vi "Add Multiple Entries.vi"(8 "error in (no error)":errorcluster, 9 "Values":variant[](array[variant]) caption="Data", 10 "Keys":string[](array[string]) caption="Names", 11 "Registry in":refnum<class "Registry.lvclass">) -> (0 "error out":errorcluster, 2 "Replaced?":bool[](array[boolean]), 3 "Registry out":refnum<class "Registry.lvclass">)   [LabVIEW 2020, in "BCI-1553 API.lvlib" / "Registry.lvlib" / "Registry.lvclass"]
doc: "Adds multiple Key/Value pairs to the Registry."
uses:
  Registry.lvclass
  Registry.lvclass/Registry.ctl
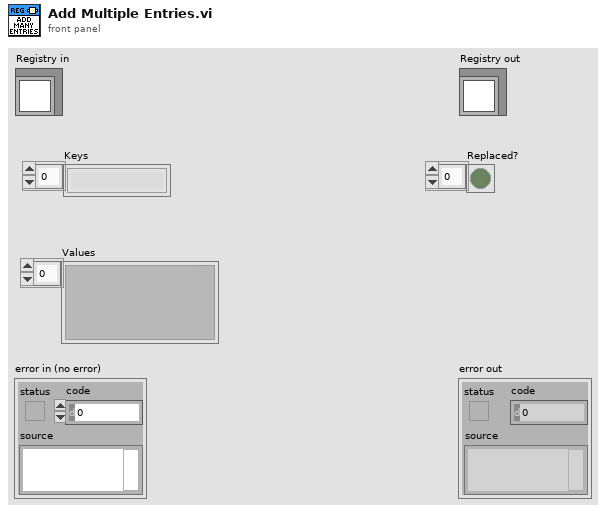
[diagram p1: front panel]
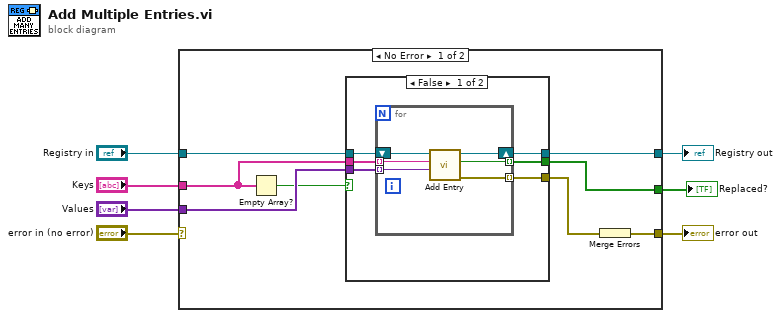
[diagram p0: block diagram]
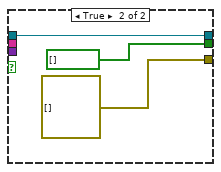
[diagram p2: hidden frame]
diagram:
  n1 = case shown="No Error" "error in (no error)" {
    selector: "error in (no error)" -> [_ w32]
    tunnel: [w10 w32] -> w6
    tunnel: [w14 w31] -> w4
    tunnel: "Registry in" -> [w15 w31]
    tunnel: "Keys" -> [w9 _]
    tunnel: "Values" -> [w13 _]
    tunnel: [w12 _] -> w1
    frame No Error {
      n2 = Empty Array?(array=w9) -> (empty?=w8:bool)
      n3 = case shown="False" w8 {
        tunnel: w15 -> [w21 w30]
        tunnel: [w20 w30] -> w14
        tunnel: w9 -> [w19 _]
        tunnel: w13 -> [w18 _]
        tunnel: [w17 bool[] []] -> w12
        tunnel: [w16 errorcluster[] []] -> w11
        frame False {
          n4 = for {
            tunnel: w19 -> [w25] mode=indexing
            tunnel: w18 -> [w24] mode=indexing
            tunnel: [w23] -> w17 mode=indexing
            shift-right: [w26] -> w20
            shift-left: w21 -> [w27]
            tunnel: [w22] -> w16 mode=indexing
            n5 = call "Add Entry.vi"("Value"=w24, "Key"=w25, "Registry in"=w27) -> ("error out"=w22:errorcluster, "Replaced?"=w23:bool, "Registry out"=w26:refnum<class "Registry.lvclass">)  [unwired: 6 in]
          }
        }
        frame True {
        }
      }
      n6 = Merge Errors(w11) -> (w10:errorcluster)
    }
    frame Error {
    }
  }
  "error out" <- w6
  "Registry out" <- w4
  "Replaced?" <- w1
